vi "Pre Launch Init.vi"(11 "Core in":refnum<class "Core.lvclass">) -> (0 "error out":errorcluster, 3 "Core out":refnum<class "Core.lvclass">)   [LabVIEW 2019, in "Core.lvlib" / "Core.lvclass"]
doc: "Sends a high priority message to it's self to notify the monitor that it's spawned. If it's in the runtime environment, this message is never sent, meaning the monitor will never spawn\n\nCopyright: MGI\n\nAuthored by Derek Trepanier\nsupport@mooregoodideas.com\nwww.mooregoodideas.com\n\nCopyright (c) 2014, Moore Good Ideas, Inc.\n\nAll rights reserved.\n\nRedistribution and use in source and binary forms, with or without modification, are permitted provided that the following conditions are met:\n\n * Redistributions of source code must retain the above copyright notice, this list of conditions and the following disclaimer.\n * Redistributions in binary form must reproduce the above copyright notice, this list of conditions and the following disclaimer in the documentation and/or other materials provided with the distribution.\n * Neither the name of Moore Good Ideas, Inc. nor the names of its contributors may be used to endorse or promote products derived from this software without specific prior written permission.\n\nTHIS SOFTWARE IS PROVIDED BY THE COPYRIGHT HOLDERS AND CONTRIBUTORS \"AS IS\" AND ANY EXPRESS OR IMPLIED WARRANTIES, INCLUDING, BUT NOT LIMITED TO, THE IMPLIED WARRANTIES OF MERCHANTABILITY AND FITNESS FOR A PARTICULAR PURPOSE ARE DISCLAIMED. IN NO EVENT SHALL THE COPYRIGHT OWNER OR CONTRIBUTORS BE LIABLE FOR ANY DIRECT, INDIRECT, INCIDENTAL, SPECIAL, EXEMPLARY, OR CONSEQUENTIAL DAMAGES (INCLUDING, BUT NOT LIMITED TO, PROCUREMENT OF SUBSTITUTE GOODS OR SERVICES; LOSS OF USE, DATA, OR PROFITS; OR BUSINESS INTERRUPTION) HOWEVER CAUSED AND ON ANY THEORY OF LIABILITY, WHETHER IN CONTRACT, STRICT LIABILITY, OR TORT (INCLUDING NEGLIGENCE OR OTHERWISE) ARISING IN ANY WAY OUT OF THE USE OF THIS SOFTWARE, EVEN IF ADVISED OF THE POSSIBILITY OF SUCH DAMAGE."
uses:
  Core.lvclass
  ModuleAbstract/ModuleAbstract.lvclass
  Classes/States/MainStates/MainStates.lvclass
  C:/Projekty/_Wewnetrzne/PC_ActorFramework/07_Program/LABVIEW/02_Source/Modules/ModuleAbstract/ModuleAbstract.lvclass
  C:/Program Files (x86)/National Instruments/LabVIEW 2019/vi.lib/MGI/Monitored Actor/Monitored Actor/Monitored Actor/Monitored Actor.lvclass
  C:/Program Files (x86)/National Instruments/LabVIEW 2019/vi.lib/ActorFramework/Actor/Actor.lvclass
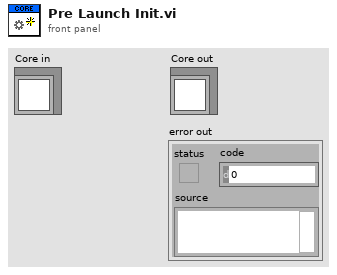
[diagram p1: front panel]
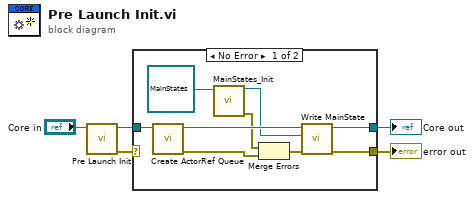
[diagram p0: block diagram]
diagram:
  n1 = call-parent "Pre Launch Init.vi"("ModuleAbstract in"="Core in") -> ("error out"=w1:errorcluster, "ModuleAbstract out"=w4:refnum<class "Core.lvclass">)  [unwired: 9 in]
  n2 = case shown="No Error" w1 {
    selector: w1 -> [_ w15]
    tunnel: w4 -> [w14 w16]
    tunnel: [w9 w16] -> w3
    tunnel: [w10 w15] -> w2
    frame No Error {
      n3 = call "Create ActorRef Queue.vi"("Core In"=w14) -> ("Error Out"=w13:errorcluster, "Core Out"=w12:refnum<class "Core.lvclass">)  [unwired: 9 in]
      n4 = call "MainStates_Init.vi"("reference in"=refnum<class "MainStates.lvclass"> refnum ("MainStates")) -> ("error out"=w8:errorcluster, "reference out"=w7:refnum<class "MainStates.lvclass">)  [unwired: 9 in]
      n5 = Merge Errors(w8, w13) -> (w11:errorcluster)
      n6 = call "Write MainState.vi"("error in (no error)"=w11, "MainStates"=w7, "ModuleAbstract in"=w12) -> ("error out"=w10:errorcluster, "ModuleAbstract out"=w9:refnum<class "Core.lvclass">)  [unwired: 7 in]
    }
    frame Error {
    }
  }
  "error out" <- w2
  "Core out" <- w3
